vi "Remove Data.vi"(6 "Unique ID":string, 7 "Remove All?":bool, 11 "Linked List Definition in":refnum<class "Linked List Definition.lvclass">) -> (3 "Linked List Definition out":refnum<class "Linked List Definition.lvclass">)   [LabVIEW 2017, in "Linked Lists.lvlib" / "Linked List Definition.lvclass"]
uses:
  <vilib>/gpm_packages/@cs/linked-list/Source/Linked List/Linked List Definition/Linked List Definition.lvclass
  <vilib>/gpm_packages/@cs/linked-list/Source/Linked List/Linked List Definition/Linked List Definition.lvclass/Linked List Definition.ctl
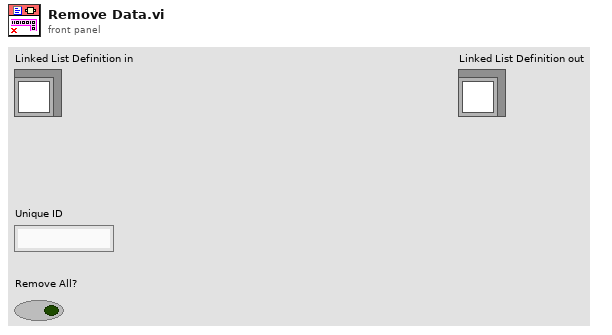
[diagram p1: front panel]
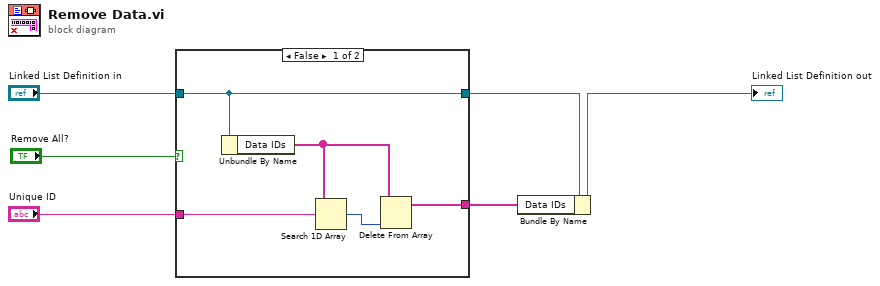
[diagram p0: block diagram]
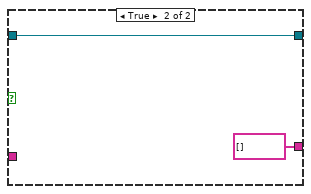
[diagram p2: hidden frame]
diagram:
  n1 = case shown="False" "Remove All?" {
    tunnel: "Unique ID" -> [w11 _]
    tunnel: [w8 string[] [] ("Data IDs")] -> w5
    tunnel: "Linked List Definition in" -> [w7 w13]
    tunnel: [w7 w13] -> w2
    frame False {
      n2 = Unbundle By Name(w7) -> ("Data IDs"=w9:string[])
      n3 = Search 1D Array(1D array=w9, element=w11) -> (index of element=w10:i32)  [unwired: 1 in]
      n4 = Delete From Array(array=w9, index=w10) -> (array with subset deleted=w8:string[])  [unwired: 1 in, 1 out]
    }
    frame True {
    }
  }
  n5 = Bundle By Name(cluster=w2, "Data IDs"=w5) -> (→"Linked List Definition out":refnum<class "Linked List Definition.lvclass">)
